vi "sorter.vi"   [LabVIEW 2015]
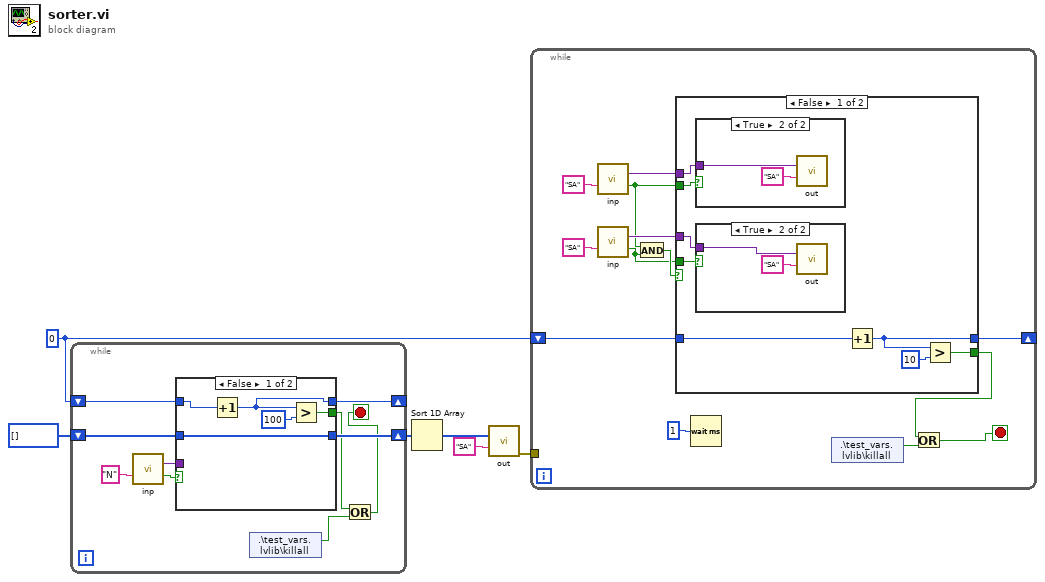
[diagram p0: block diagram]
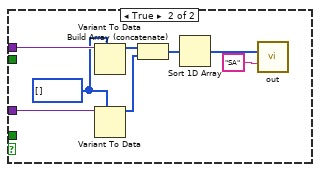
[diagram p4: hidden frame]
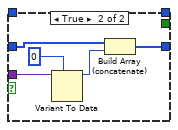
[diagram p5: hidden frame]
diagram:
  w2 = 0
  n1 = while {
    shift-right: [w13] -> w6
    shift-left: u32[] [] -> [w15]
    shift-right: [w11] -> _
    shift-left: w2 -> [w12]
    stop <- w7 stop-if-true
    n2 = call "inp.vi"("Name in"="N") -> ("OUT VARIANT"=w14:variant, "Valid data"=w10:bool)  [unwired: 12 in, 1 out]
    n3 = case shown="False" w10 {
      tunnel: w15 -> [w21 w26]
      tunnel: w14 -> [_ w24]
      tunnel: [w21 w22] -> w13
      tunnel: w12 -> [w20 _]
      tunnel: [w19 _] -> w11
      tunnel: [w17 _] -> w8
      frame False {
        n4 = Increment(x=w20) -> (x+1=w19:i32)
        n5 = Greater?(x=w19, y=100) -> (0:w17:bool)
      }
      frame True {
        n6 = Variant To Data(type=u32 0, Variant=w24) -> (data=w23:u32)  [unwired: 1 in, 1 out]
        n7 = Build Array (concatenate)(w26, w23) -> (w22:u32[])
      }
    }
    n8 = shared-variable ".\\test_vars.lvlib\\killall"() -> (w9:bool)  [unwired: 1 in, 1 out]
    n9 = Or(x=w8, y=w9) -> (x .or. y?=w7:bool)
  }
  n10 = Sort 1D Array(array=w6) -> (sorted array=w5:u32[])
  n11 = call "out.vi"("IN VARIANT"=w5, "Name in"="SA") -> ("error out"=w1:errorcluster)  [unwired: 12 in, 1 out]
  n12 = while {
    shift-right: [w38] -> _
    shift-left: w2 -> [w39]
    tunnel: w1 -> [_]
    stop <- w27 stop-if-true
    n13 = call "inp.vi"("Name in"="SA") -> ("OUT VARIANT"=w37:variant, "Valid data"=w32:bool)  [unwired: 12 in, 1 out]
    n14 = call "inp.vi"("Name in"="SA") -> ("OUT VARIANT"=w33:variant, "Valid data"=w31:bool)  [unwired: 12 in, 1 out]
    n15 = And(x=w32, y=w31) -> (x .and. y?=w34:bool)
    n16 = case shown="False" w34 {
      tunnel: w37 -> [w41 w59]
      tunnel: w39 -> [w47 _]
      tunnel: [w46 _] -> w38
      tunnel: [w44 _] -> w28
      tunnel: w33 -> [w43 w58]
      tunnel: w31 -> [w42 _]
      tunnel: w32 -> [w40 _]
      frame False {
        n17 = case shown="True" w40 {
          tunnel: w41 -> [_ w48]
          frame False {
          }
          frame True {
            n18 = call "out.vi"("IN VARIANT"=w48, "Name in"="SA") -> ()  [unwired: 12 in, 2 out]
          }
        }
        n19 = case shown="True" w42 {
          tunnel: w43 -> [_ w50]
          frame False {
          }
          frame True {
            n20 = call "out.vi"("IN VARIANT"=w50, "Name in"="SA") -> ()  [unwired: 12 in, 2 out]
          }
        }
        n21 = Increment(x=w47) -> (x+1=w46:i32)
        n22 = Greater?(x=w46, y=10) -> (0:w44:bool)
      }
      frame True {
        w53 = u32[] []
        n23 = Variant To Data(type=w53, Variant=w59) -> (data=w57:u32[])  [unwired: 1 in, 1 out]
        n24 = Variant To Data(type=w53, Variant=w58) -> (data=w56:u32[])  [unwired: 1 in, 1 out]
        n25 = Build Array (concatenate)(w57, w56) -> (w52:u32[])
        n26 = Sort 1D Array(array=w52) -> (sorted array=w54:u32[])
        n27 = call "out.vi"("IN VARIANT"=w54, "Name in"="SA") -> ()  [unwired: 12 in, 2 out]
      }
    }
    n28 = Wait (ms)(milliseconds to wait=u32 1) -> ()  [unwired: 1 out]
    n29 = shared-variable ".\\test_vars.lvlib\\killall"() -> (w29:bool)  [unwired: 1 in, 1 out]
    n30 = Or(x=w28, y=w29) -> (x .or. y?=w27:bool)
  }
